vi "Envio-Variant.vi"() -> ()   [LabVIEW 2016]
panel:
  in  "Numeric Control 2":i8
  out "variant":variant
  in  "String":string
  in  "Boolean":bool
  in  "Numeric Control":dbl
  in  "Detener":bool
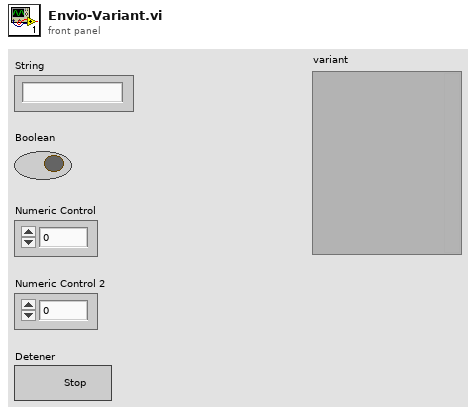
[diagram p1: front panel]
types:
  T1 = enum16{"Read", "Write", "ReadWrite", "BufferedRead", "BufferedReadWrite"}
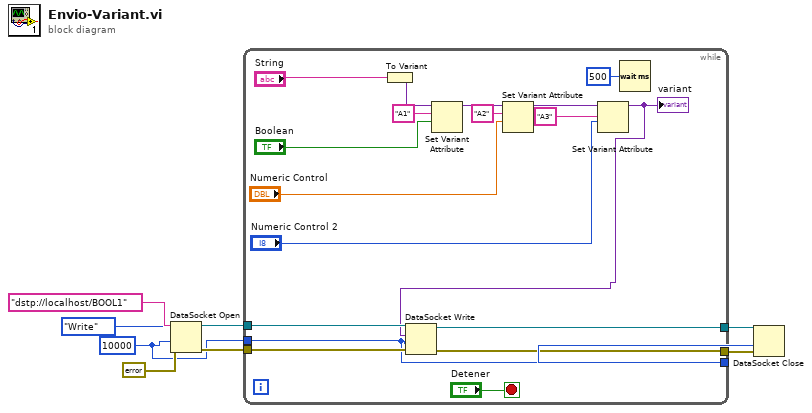
[diagram p0: block diagram]
diagram:
  w1 = 10000 ("ms timeout (10000)")
  n1 = DataSocket Open(8:errorcluster {"status"=FALSE, "code"=0, "source"=""} ("error in (no error)"), 9:w1, 10:T1."Write" ("mode"), 11:"dstp://localhost/BOOL1" ("connection in")) -> (0:w6:errorcluster, 3:w5:refnum<k13>)
  n2 = while {
    tunnel: w6 -> [w25]
    tunnel: w5 -> [w24]
    tunnel: [w23] -> w4
    tunnel: [w22] -> w3
    tunnel: w1 -> [w21]
    tunnel: [w21] -> w2
    stop <- "Detener" stop-if-true
    n3 = To Variant(anything="String") -> (Variant=w20:variant)
    n4 = Set Variant Attribute(Variant=w20, name="A1", value="Boolean") -> (Variant out=w17:variant)  [unwired: 1 in, 2 out]
    n5 = Set Variant Attribute(Variant=w17, name="A2", value="Numeric Control") -> (Variant out=w15:variant)  [unwired: 1 in, 2 out]
    n6 = Set Variant Attribute(Variant=w15, name="A3", value="Numeric Control 2") -> (Variant out=w10:variant)  [unwired: 1 in, 2 out]
    "variant" <- w10
    n7 = DataSocket Write(8:w25, 9:w21, 10:w10, 11:w24) -> (0:w22:errorcluster, 3:w23:refnum<k13>)  [unwired: 1 out]
    n8 = Wait (ms)(milliseconds to wait=u32 500) -> ()  [unwired: 1 out]
  }
  n9 = DataSocket Close(8:w3, 9:w2, 11:w4) -> ()  [unwired: 2 out]
